vi "PM_Close.vi"(0 "instrument handle":refnum<visa-resource-name>, 7 "Sensor":string, 11 "error in (no error)":errorcluster {"code" format="%.0x"}) -> (8 "Sensor 2":string, 15 "error out":errorcluster)   [LabVIEW 2018]
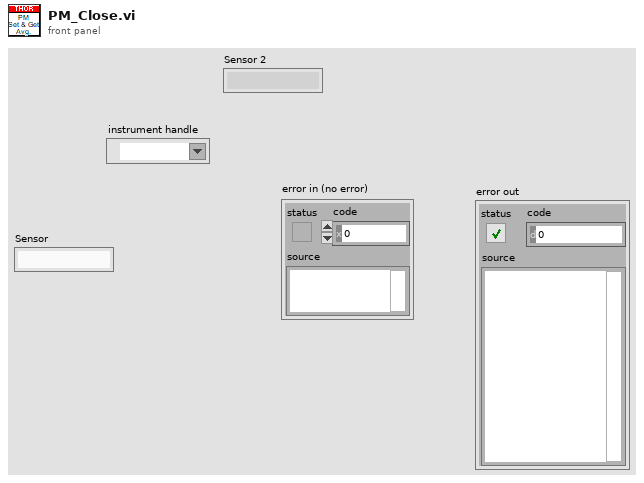
[diagram p1: front panel]
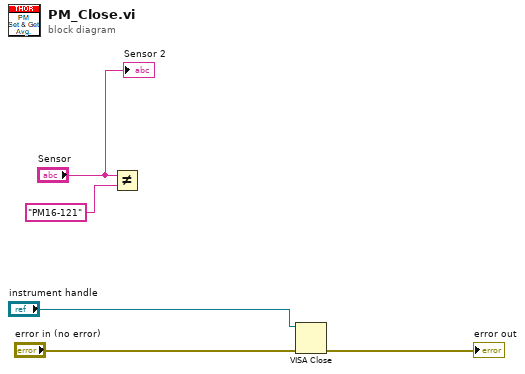
[diagram p0: block diagram]
diagram:
  n1 = Not Equal?(x="Sensor", y="PM16-121") -> ()  [unwired: 1 out]
  n2 = VISA Close(VISA resource name="instrument handle", error in (no error)="error in (no error)") -> (error out=→"error out":errorcluster)
  "Sensor 2" <- "Sensor"
